vi "Determining_Change_RunNumber.vi"(8 "error in":errorcluster, 11 "Run Folder Parent Directory":path) -> (0 "error out":errorcluster, 1 "Array":dbl[](array[numeric]), 2 "String":string, 3 "path out":path, 4 "Proposed Run Number":i32, 5 "T button?":bool)   [LabVIEW 2019]
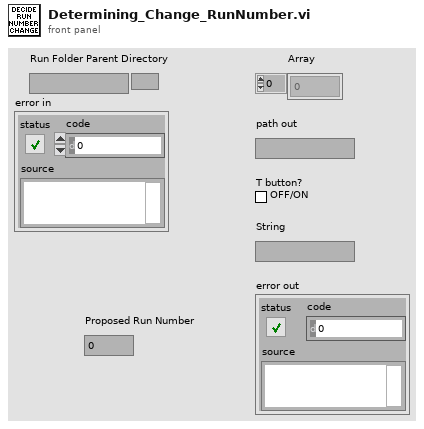
[diagram p1: front panel]
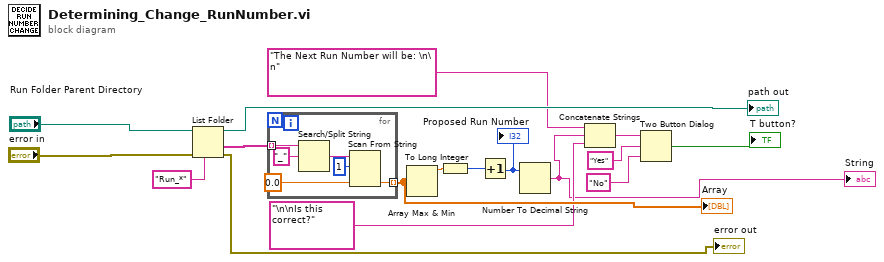
[diagram p0: block diagram]
diagram:
  n1 = List Folder(path="Run Folder Parent Directory", pattern="Run_*", error in="error in") -> (path out=→"path out":path, folder names=w7:string[], error out=→"error out":errorcluster)  [unwired: 1 in, 1 out]
  n2 = for {
    tunnel: w7 -> [w23] mode=indexing
    tunnel: [w18] -> w13 mode=indexing
    n3 = Search/Split String(string=w23, search string/char (-)="_") -> (match + rest of string=w21:string)  [unwired: 1 in, 2 out]
    n4 = Scan From String(input string=w21, initial scan location=u32 1, default 1=0.0 ("default value 1")) -> (output 1=w18:dbl)  [unwired: 2 in, 3 out]
  }
  "Array" <- w13
  n5 = Array Max & Min(array=w13) -> (max value=w4:dbl)  [unwired: 3 out]
  n6 = To Long Integer(number=w4) -> (32bit integer=w1:i32)
  n7 = Increment(x=w1) -> (x+1=w2:i32)
  "Proposed Run Number" <- w2
  n8 = Number To Decimal String(number=w2) -> (decimal integer string=w3:string)  [unwired: 1 in]
  "String" <- w3
  n9 = Concatenate Strings("The Next Run Number will be: \n\n" ("string"), w3, "\n\nIs this correct?" ("string")) -> (w12:string)
  n10 = Two Button Dialog(message=w12, 1:"No" ("F button name (\"Cancel\")"), 2:"Yes" ("T button name (\"OK\")")) -> (T button?=→"T button?":bool)
